vi "get piece from floor.vi"() -> ()   [LabVIEW 2018]
uses:
  vision/Vision info.vi
panel:
  in  "base":i32(slide) scale=-125.0..125.0
  out "Type":enum16{"Z", "I", "O", "S", "L", "J", "T", "N"}(ring)
  out "angel":dbl
  in  "grip":bool
  in  "camera mode":bool
  in  "z1":dbl
  in  "z2":dbl
  in  "step":dbl
  in  "speed 1":i32
  in  "y_plus":dbl
  in  "take":bool
  in  "x_plus":dbl
  in  "move":bool
  out "_x":dbl
  out "_y":dbl
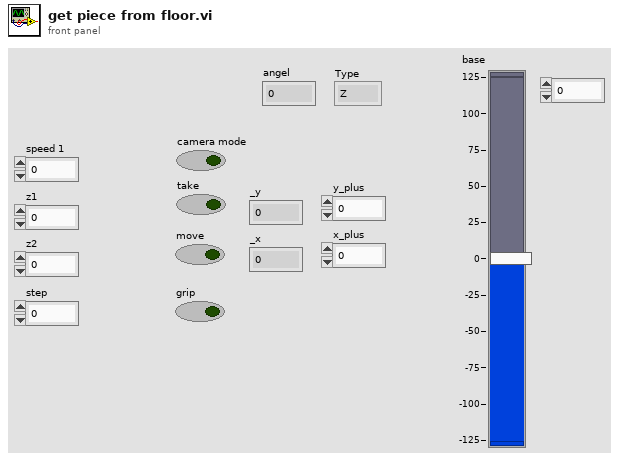
[diagram p1: front panel]
types:
  T1 = enum16{"shoulder", "elbow", "wrist", "base", "gripper"}
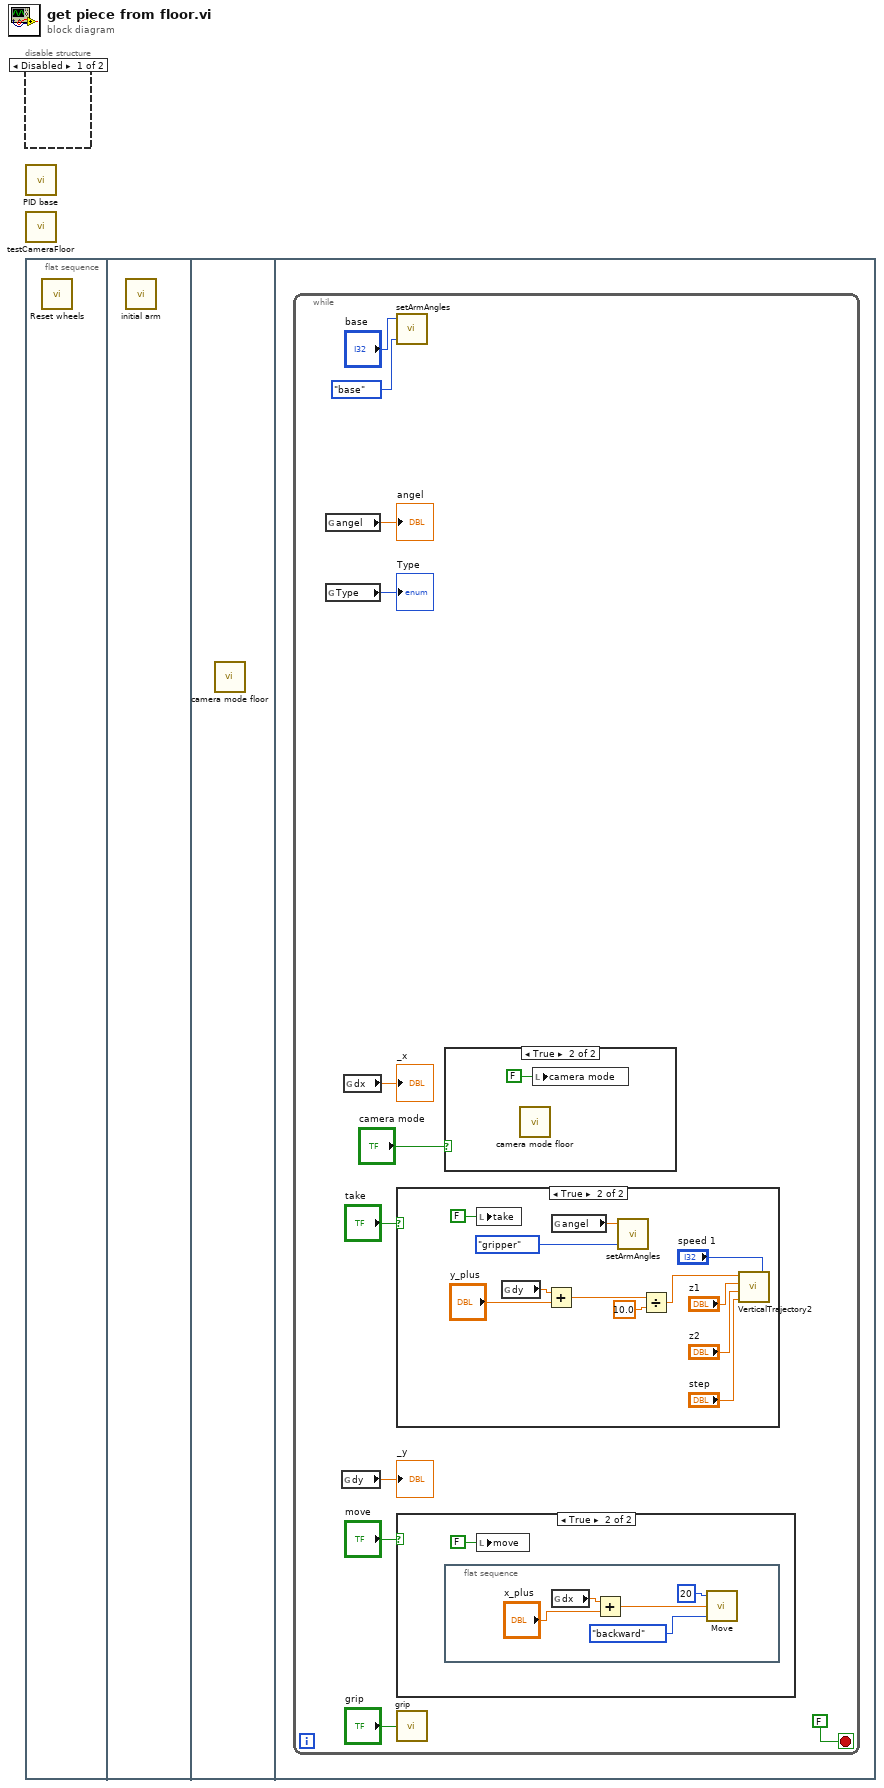
[diagram p0: block diagram]
diagram:
  n1 = disable-structure shown="Disabled" {
    frame Disabled {
    }
    frame Enabled {
    }
  }
  n2 = call "PID base.vi"() -> ()  [unwired: 12 in]
  n3 = call "testCameraFloor.vi"() -> ()  [unwired: 12 in]
  n4 = flat-sequence {
    frame #0 {
      n5 = call "Reset wheels.vi"() -> ()  [unwired: 12 in]
    }
    frame #1 {
      n6 = call "initial arm.vi"() -> ()  [unwired: 12 in]
    }
    frame #2 {
      n7 = call "camera mode floor.vi"() -> ()  [unwired: 12 in]
    }
    frame #3 {
      n8 = while {
        stop <- FALSE stop-if-true
        n9 = global read "Vision info.vi" "angel"() -> (→"angel":dbl)
        n10 = global read "Vision info.vi" "Type"() -> (→"Type":enum16{"Z", "I", "O", "S", "L", "J", "T", "N"})
        n11 = global read "Vision info.vi" "dy"() -> (→"_y":dbl)
        n12 = global read "Vision info.vi" "dx"() -> (→"_x":dbl)
        n13 = call "setArmAngles.vi"("Enum"=enum16{"shoulder", "elbow", "wrist", "base"}."base", "angle"="base") -> ()  [unwired: 2 in]
        n14 = case shown="True" "take" {
          frame False {
          }
          frame True {
            n15 = local write "take"(FALSE ("take")) -> ()
            n16 = global read "Vision info.vi" "dy"() -> (w20:dbl)
            n17 = Add(x=w20, y="y_plus") -> (x+y=w23:dbl)
            n18 = global read "Vision info.vi" "angel"() -> (w19:dbl)
            n19 = call "setArmAngles.vi"("Enum"=T1."gripper", "angle"=w19) -> ()  [unwired: 2 in]
            n20 = Divide(x=w23, y=10.0) -> (x/y=w21:dbl)
            n21 = call "VerticalTrajectory2.vi"("speed 1"="speed 1", "step"="step", "z2"="z2", "z1"="z1", "x"=w21) -> ()  [unwired: 3 in]
          }
        }
        n22 = case shown="True" "move" {
          frame False {
          }
          frame True {
            n23 = flat-sequence {
              frame #0 {
                n24 = global read "Vision info.vi" "dx"() -> (w13:dbl)
                n25 = Add(x=w13, y="x_plus") -> (x+y=w14:dbl)
                n26 = call "Move.vi"("Enum"=enum16{"forward", "backward", "left", "right"}."backward", "distance"=w14, "speed"=20) -> ()  [unwired: 1 in]
              }
            }
            n27 = local write "move"(FALSE ("move")) -> ()
          }
        }
        n28 = call "grip.vi"("grip"="grip") -> ()
        n29 = case shown="True" "camera mode" {
          frame False {
          }
          frame True {
            n30 = call "camera mode floor.vi"() -> ()  [unwired: 12 in]
            n31 = local write "camera mode"(FALSE ("camera mode")) -> ()
          }
        }
      }
    }
  }
